vi "ReadResponseFromBrooksMFC.vi"(8 "error in":errorcluster, 11 "Brooks MFC in":refnum<class "Brooks MFC.lvclass">) -> (0 "error out":errorcluster, 1 "Data":u8[](array[numeric])=[17, 17, 136, 232, 65] format="%.0x", 2 "Command":u8=1 format="%.0x", 3 "Brooks MFC out":refnum<class "Brooks MFC.lvclass">, 4 "device type":u8, 5 "tag ID":u32)   [LabVIEW 2016, in "Brooks MFC.lvclass"]
uses:
  Brooks MFC.lvclass
  Brooks MFC.lvclass/Brooks MFC.ctl
panel:
  out "return count":u32
  out "Status Byte":u8[](array[numeric]) format="%x"
  out "Bytecount":u8=7 format="%.0x"
  out "checksum":bool=TRUE
  out "acknowledge":bool=TRUE
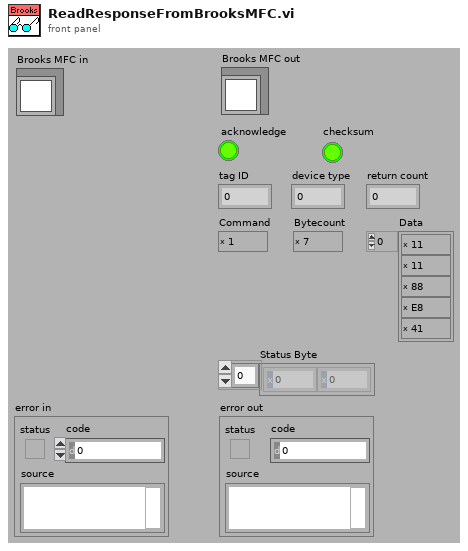
[diagram p1: front panel]
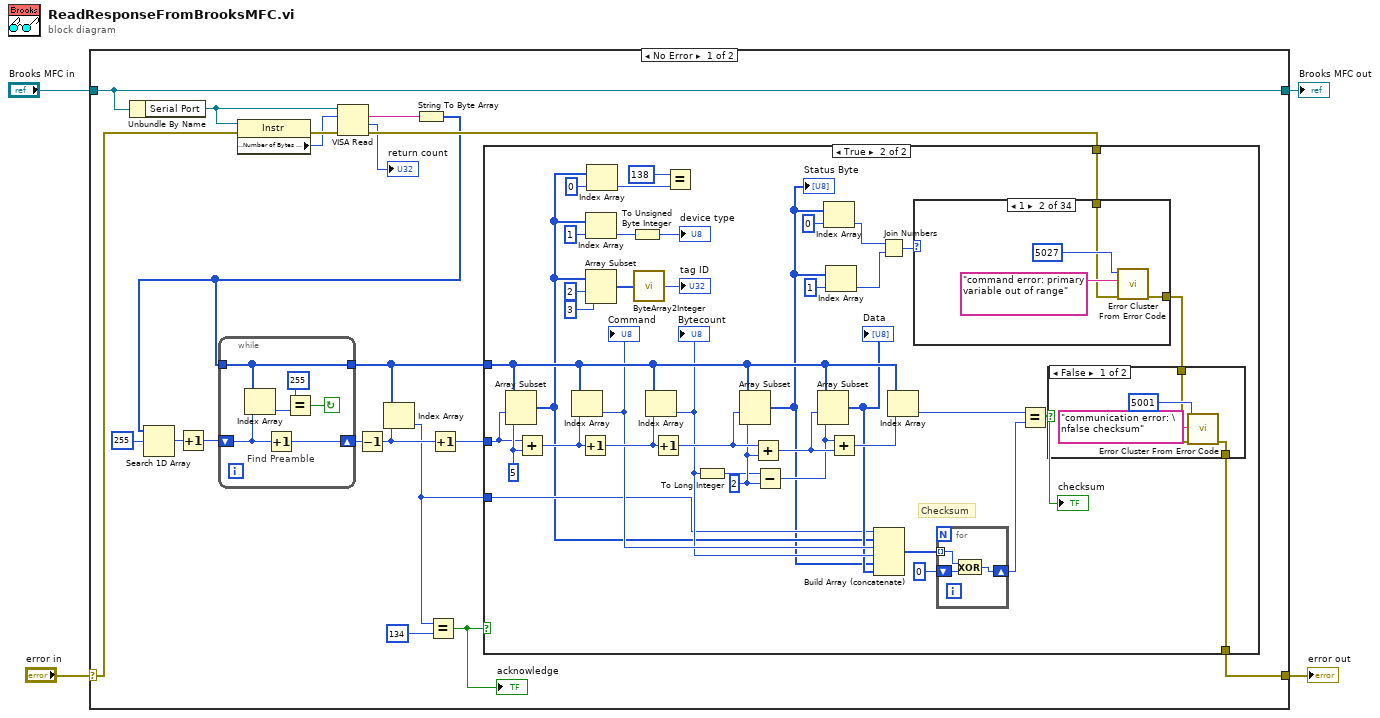
[diagram p0: block diagram]
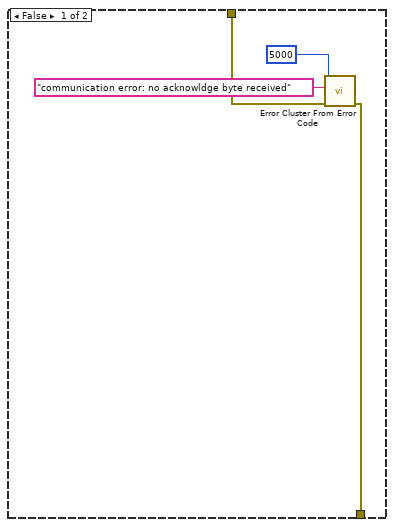
[diagram p2: hidden frame]
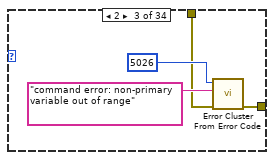
[diagram p4: hidden frame]
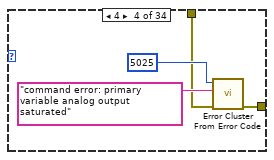
[diagram p5: hidden frame]
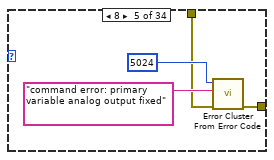
[diagram p6: hidden frame]
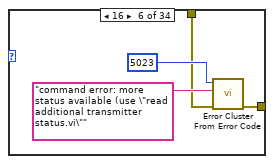
[diagram p7: hidden frame]
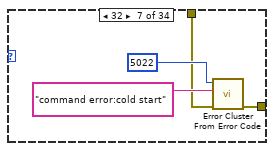
[diagram p8: hidden frame]
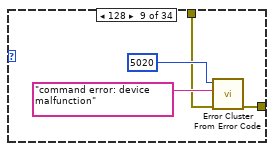
[diagram p10: hidden frame]
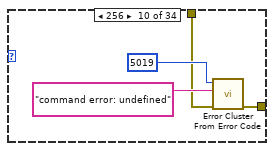
[diagram p11: hidden frame]
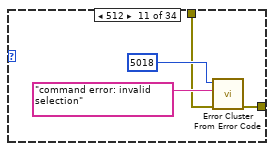
[diagram p12: hidden frame]
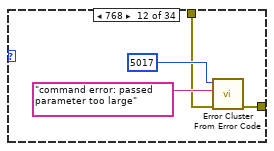
[diagram p13: hidden frame]
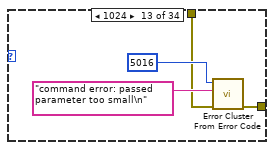
[diagram p14: hidden frame]
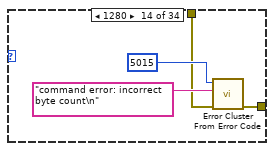
[diagram p15: hidden frame]
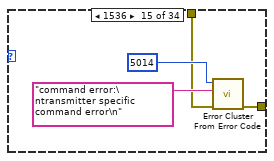
[diagram p16: hidden frame]
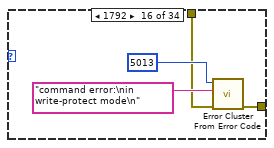
[diagram p17: hidden frame]
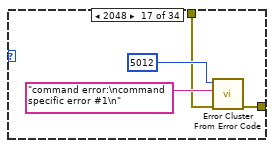
[diagram p18: hidden frame]
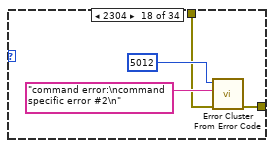
[diagram p19: hidden frame]
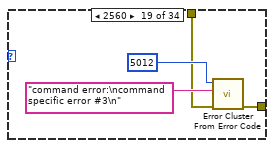
[diagram p20: hidden frame]
diagram:
  n1 = case shown="No Error" "error in" {
    selector: "error in" -> [w6 w214]
    tunnel: "Brooks MFC in" -> [w7 w213]
    tunnel: [w9 w214] -> w2
    tunnel: [w7 w213] -> w1
    frame No Error {
      n2 = Unbundle By Name(w7) -> ("Serial Port"=w8:refnum<visa-resource-name>)
      n3 = property class="Instr"(reference=w8, error in=w6) -> (error out=w13:errorcluster, "Serial Settings:Number of Bytes at Serial Port"=w12:u32)  [unwired: 1 out]
      n4 = VISA Read(VISA resource name=w8, byte count=w12, error in (no error)=w13) -> (read buffer=w14:string, return count=→"return count":u32, error out=w11:errorcluster)  [unwired: 1 out]
      n5 = String To Byte Array(string=w14) -> (unsigned byte array=w10:u8[])
      n6 = Search 1D Array(1D array=w10, element=u8 255) -> (index of element=w16:i32)  [unwired: 1 in]
      n7 = Increment(x=w16) -> (x+1=w18:i32)
      n8 = while {
        tunnel: [w26] -> w22
        shift-left: w18 -> [w29]
        shift-right: [w30] -> w20
        tunnel: w10 -> [w26]
        stop <- w25 continue-if-true
        # "Find Preamble"
        n9 = Index Array(array=w26, index=w29) -> (element=w28:u8)
        n10 = Increment(x=w29) -> (x+1=w30:i32)
        n11 = Equal?(x=u8 255, y=w28) -> (x = y?=w25:bool)
      }
      n12 = Decrement(x=w20) -> (x-1=w24:i32)
      n13 = Index Array(array=w22, index=w24) -> (element=w23:u8)
      n14 = Equal?(x=w23, y=134) -> (x = y?=w19:bool)
      "acknowledge" <- w19
      n15 = Increment(x=w24) -> (x+1=w21:i32)
      n16 = case shown="True" w19 {
        tunnel: w21 -> [_ w73]
        tunnel: w22 -> [_ w68]
        tunnel: w23 -> [_ w60]
        tunnel: w11 -> [w32 w37]
        tunnel: [w31 w35] -> w9
        frame False {
          n17 = call <vilib>:"Error Cluster From Error Code.vi"("error in (no error)"=w32, "error message (\"\")"="communication error: no acknowldge byte received", "error code (0)"=5000) -> ("error out"=w31:errorcluster)  [unwired: 6 in]
        }
        frame True {
          w69 = 2 ("Array Length")
          w74 = 5 ("Array Length")
          # "Checksum"
          n18 = Array Subset(array=w68, index=w73, length=w74) -> (w52:u8[])
          n19 = Add(x=w73, y=w74) -> (x+y=w72:i32)
          n20 = Index Array(array=w68, index=w72) -> (element=w63:u8)
          "Command" <- w63
          n21 = Increment(x=w72) -> (x+1=w71:i32)
          n22 = Index Array(array=w52, index=1) -> (element=w47:u8)
          n23 = Array Subset(array=w52, index=2, length=3) -> (w49:u8[])
          n24 = Index Array(array=w52, index=0) -> (element=w45:u8)
          n25 = To Unsigned Byte Integer(number=w47) -> (unsigned 8bit integer=→"device type":u8)
          n26 = call "ByteArray2Integer.vi"("Byte Array"=w49) -> ("Integer"=→"tag ID":u32)
          n27 = Index Array(array=w68, index=w71) -> (element=w62:u8)
          "Bytecount" <- w62
          n28 = Increment(x=w71) -> (x+1=w70:i32)
          n29 = Equal?(x=u8 138, y=w45) -> ()  [unwired: 1 out]
          n30 = To Long Integer(number=w62) -> (32bit integer=w59:i32)
          n31 = Array Subset(array=w68, index=w70, length=w69) -> (w41:u8[])
          "Status Byte" <- w41
          n32 = Add(x=w70, y=w69) -> (x+y=w66:i32)
          n33 = Subtract(x=w59, y=w69) -> (x-y=w65:i32)
          n34 = Array Subset(array=w68, index=w66, length=w65) -> (w61:u8[])
          "Data" <- w61
          n35 = Index Array(array=w41, index=0) -> (element=w39:u8)
          n36 = Index Array(array=w41, index=1) -> (element=w40:u8)
          n37 = Add(x=w65, y=w66) -> (x+y=w64:i32)
          n38 = Build Array (concatenate)(w60, w52, w63, w62, w41, w61) -> (w57:u8[])
          n39 = Join Numbers(hi=w39, lo=w40) -> ((hi.lo)=w38:u16)
          n40 = Index Array(array=w68, index=w64) -> (element=w67:u8)
          n41 = case shown="1" w38 {
            tunnel: w37 -> [w75 w77 w81 w85 w89 w93 w97 w100 w102 w106 w110 w114 w118 w122 w126 w130 w134 w138 w142 w146 w150 w154 w158 w162 w166 w170 w174 w178 w182 w186 w190 w194 w198 w202]
            tunnel: [w75 w76 w80 w84 w88 w92 w96 w100 w101 w105 w109 w113 w117 w121 w125 w129 w133 w137 w141 w145 w149 w153 w157 w161 w165 w169 w173 w177 w181 w185 w189 w193 w197 w201] -> w36
            frame 0, Default {
            }
            frame 1 {
              n42 = call <vilib>:"Error Cluster From Error Code.vi"("error in (no error)"=w77, "error message (\"\")"="command error: primary variable out of range" ("error message (\"\")"), "error code (0)"=5027) -> ("error out"=w76:errorcluster)  [unwired: 6 in]
            }
            frame 2 {
              n43 = call <vilib>:"Error Cluster From Error Code.vi"("error in (no error)"=w81, "error message (\"\")"="command error: non-primary variable out of range" ("error message (\"\")"), "error code (0)"=5026) -> ("error out"=w80:errorcluster)  [unwired: 6 in]
            }
            frame 4 {
              n44 = call <vilib>:"Error Cluster From Error Code.vi"("error in (no error)"=w85, "error message (\"\")"="command error: primary variable analog output saturated" ("error message (\"\")"), "error code (0)"=5025) -> ("error out"=w84:errorcluster)  [unwired: 6 in]
            }
            frame 8 {
              n45 = call <vilib>:"Error Cluster From Error Code.vi"("error in (no error)"=w89, "error message (\"\")"="command error: primary variable analog output fixed" ("error message (\"\")"), "error code (0)"=5024) -> ("error out"=w88:errorcluster)  [unwired: 6 in]
            }
            frame 16 {
              n46 = call <vilib>:"Error Cluster From Error Code.vi"("error in (no error)"=w93, "error message (\"\")"="command error: more status available (use \"read additional transmitter status.vi\"" ("error message (\"\")"), "error code (0)"=5023) -> ("error out"=w92:errorcluster)  [unwired: 6 in]
            }
            frame 32 {
              n47 = call <vilib>:"Error Cluster From Error Code.vi"("error in (no error)"=w97, "error message (\"\")"="command error:cold start" ("error message (\"\")"), "error code (0)"=5022) -> ("error out"=w96:errorcluster)  [unwired: 6 in]
            }
            frame 64 {
            }
            frame 128 {
              n48 = call <vilib>:"Error Cluster From Error Code.vi"("error in (no error)"=w102, "error message (\"\")"="command error: device malfunction" ("error message (\"\")"), "error code (0)"=5020) -> ("error out"=w101:errorcluster)  [unwired: 6 in]
            }
            frame 256 {
              n49 = call <vilib>:"Error Cluster From Error Code.vi"("error in (no error)"=w106, "error message (\"\")"="command error: undefined" ("error message (\"\")"), "error code (0)"=5019) -> ("error out"=w105:errorcluster)  [unwired: 6 in]
            }
            frame 512 {
              n50 = call <vilib>:"Error Cluster From Error Code.vi"("error in (no error)"=w110, "error message (\"\")"="command error: invalid selection" ("error message (\"\")"), "error code (0)"=5018) -> ("error out"=w109:errorcluster)  [unwired: 6 in]
            }
            frame 768 {
              n51 = call <vilib>:"Error Cluster From Error Code.vi"("error in (no error)"=w114, "error message (\"\")"="command error: passed parameter too large" ("error message (\"\")"), "error code (0)"=5017) -> ("error out"=w113:errorcluster)  [unwired: 6 in]
            }
            frame 1024 {
              n52 = call <vilib>:"Error Cluster From Error Code.vi"("error in (no error)"=w118, "error message (\"\")"="command error: passed parameter too small\n" ("error message (\"\")"), "error code (0)"=5016) -> ("error out"=w117:errorcluster)  [unwired: 6 in]
            }
            frame 1280 {
              n53 = call <vilib>:"Error Cluster From Error Code.vi"("error in (no error)"=w122, "error message (\"\")"="command error: incorrect byte count\n" ("error message (\"\")"), "error code (0)"=5015) -> ("error out"=w121:errorcluster)  [unwired: 6 in]
            }
            frame 1536 {
              n54 = call <vilib>:"Error Cluster From Error Code.vi"("error in (no error)"=w126, "error message (\"\")"="command error:\ntransmitter specific command error\n" ("error message (\"\")"), "error code (0)"=5014) -> ("error out"=w125:errorcluster)  [unwired: 6 in]
            }
            frame 1792 {
              n55 = call <vilib>:"Error Cluster From Error Code.vi"("error in (no error)"=w130, "error message (\"\")"="command error:\nin write-protect mode\n" ("error message (\"\")"), "error code (0)"=5013) -> ("error out"=w129:errorcluster)  [unwired: 6 in]
            }
            frame 2048 {
              n56 = call <vilib>:"Error Cluster From Error Code.vi"("error in (no error)"=w134, "error message (\"\")"="command error:\ncommand specific error #1\n" ("error message (\"\")"), "error code (0)"=5012) -> ("error out"=w133:errorcluster)  [unwired: 6 in]
            }
            frame 2304 {
              n57 = call <vilib>:"Error Cluster From Error Code.vi"("error in (no error)"=w138, "error message (\"\")"="command error:\ncommand specific error #2\n" ("error message (\"\")"), "error code (0)"=5012) -> ("error out"=w137:errorcluster)  [unwired: 6 in]
            }
            frame 2560 {
              n58 = call <vilib>:"Error Cluster From Error Code.vi"("error in (no error)"=w142, "error message (\"\")"="command error:\ncommand specific error #3\n" ("error message (\"\")"), "error code (0)"=5012) -> ("error out"=w141:errorcluster)  [unwired: 6 in]
            }
            frame 2816 {
              n59 = call <vilib>:"Error Cluster From Error Code.vi"("error in (no error)"=w146, "error message (\"\")"="command error:\ncommand specific error #4\n" ("error message (\"\")"), "error code (0)"=5012) -> ("error out"=w145:errorcluster)  [unwired: 6 in]
            }
            frame 3072 {
              n60 = call <vilib>:"Error Cluster From Error Code.vi"("error in (no error)"=w150, "error message (\"\")"="command error:\ncommand specific error #5\n" ("error message (\"\")"), "error code (0)"=5012) -> ("error out"=w149:errorcluster)  [unwired: 6 in]
            }
            frame 3328 {
              n61 = call <vilib>:"Error Cluster From Error Code.vi"("error in (no error)"=w154, "error message (\"\")"="command error:\ncommand specific error #6\n" ("error message (\"\")"), "error code (0)"=5012) -> ("error out"=w153:errorcluster)  [unwired: 6 in]
            }
            frame 3584 {
              n62 = call <vilib>:"Error Cluster From Error Code.vi"("error in (no error)"=w158, "error message (\"\")"="command error:\ncommand specific error #7\n" ("error message (\"\")"), "error code (0)"=5012) -> ("error out"=w157:errorcluster)  [unwired: 6 in]
            }
            frame 3840 {
              n63 = call <vilib>:"Error Cluster From Error Code.vi"("error in (no error)"=w162, "error message (\"\")"="command error:\ncommand specific error #8\n" ("error message (\"\")"), "error code (0)"=5012) -> ("error out"=w161:errorcluster)  [unwired: 6 in]
            }
            frame 4096 {
              n64 = call <vilib>:"Error Cluster From Error Code.vi"("error in (no error)"=w166, "error message (\"\")"="command error:\naccess restricted\n" ("error message (\"\")"), "error code (0)"=5011) -> ("error out"=w165:errorcluster)  [unwired: 6 in]
            }
            frame 8192 {
              n65 = call <vilib>:"Error Cluster From Error Code.vi"("error in (no error)"=w170, "error message (\"\")"="command error:\ndevice is busy" ("error message (\"\")"), "error code (0)"=5010) -> ("error out"=w169:errorcluster)  [unwired: 6 in]
            }
            frame 16384 {
              n66 = call <vilib>:"Error Cluster From Error Code.vi"("error in (no error)"=w174, "error message (\"\")"="command error:\ncommand not implemented\n" ("error message (\"\")"), "error code (0)"=5009) -> ("error out"=w173:errorcluster)  [unwired: 6 in]
            }
            frame 33024 {
              n67 = call <vilib>:"Error Cluster From Error Code.vi"("error in (no error)"=w178, "error message (\"\")"="communication error:\nnot defined\n" ("error message (\"\")"), "error code (0)"=5008) -> ("error out"=w177:errorcluster)  [unwired: 6 in]
            }
            frame 33280 {
              n68 = call <vilib>:"Error Cluster From Error Code.vi"("error in (no error)"=w182, "error message (\"\")"="communication error:\nrx buffer overflow error\n" ("error message (\"\")"), "error code (0)"=5007) -> ("error out"=w181:errorcluster)  [unwired: 6 in]
            }
            frame 33792 {
              n69 = call <vilib>:"Error Cluster From Error Code.vi"("error in (no error)"=w186, "error message (\"\")"="communication error:\nreserved error\n" ("error message (\"\")"), "error code (0)"=5006) -> ("error out"=w185:errorcluster)  [unwired: 6 in]
            }
            frame 34816 {
              n70 = call <vilib>:"Error Cluster From Error Code.vi"("error in (no error)"=w190, "error message (\"\")"="communication error:\nchecksum error\n" ("error message (\"\")"), "error code (0)"=5005) -> ("error out"=w189:errorcluster)  [unwired: 6 in]
            }
            frame 36864 {
              n71 = call <vilib>:"Error Cluster From Error Code.vi"("error in (no error)"=w194, "error message (\"\")"="communication error:\nframing error\n" ("error message (\"\")"), "error code (0)"=5004) -> ("error out"=w193:errorcluster)  [unwired: 6 in]
            }
            frame 40960 {
              n72 = call <vilib>:"Error Cluster From Error Code.vi"("error in (no error)"=w198, "error message (\"\")"="communication error:\noverrun error\n" ("error message (\"\")"), "error code (0)"=5003) -> ("error out"=w197:errorcluster)  [unwired: 6 in]
            }
            frame 49152 {
              n73 = call <vilib>:"Error Cluster From Error Code.vi"("error in (no error)"=w202, "error message (\"\")"="communication error:\nparity error\n" ("error message (\"\")"), "error code (0)"=5002) -> ("error out"=w201:errorcluster)  [unwired: 6 in]
            }
          }
          n74 = for {
            shift-right: [w206] -> w56
            shift-left: u8 0 -> [w207]
            tunnel: w57 -> [w205] mode=indexing
            n75 = Exclusive Or(1:w207, 2:w205) -> (0:w206:u8)
          }
          n76 = Equal?(x=w67, y=w56) -> (x = y?=w55:bool)
          "checksum" <- w55
          n77 = case shown="False" w55 {
            tunnel: w36 -> [w209 w212]
            tunnel: [w208 w212] -> w35
            frame False {
              n78 = call <vilib>:"Error Cluster From Error Code.vi"("error in (no error)"=w209, "error message (\"\")"="communication error: \nfalse checksum", "error code (0)"=5001) -> ("error out"=w208:errorcluster)  [unwired: 6 in]
            }
            frame True {
            }
          }
        }
      }
    }
    frame Error {
    }
  }
  "error out" <- w2
  "Brooks MFC out" <- w1
